vi "Send SetSlitwidth.vi"(7 "Message Priority (Normal)":T2=enum."Normal", 8 "error in (no error)":errorcluster, 9 "Slitwidth":u16, 10 "Slit":T1(ring), 11 "Message Enqueuer":refnum<class "Message Enqueuer.lvclass">) -> (0 "error out":errorcluster, 3 "Message Enqueuer out":refnum<class "Message Enqueuer.lvclass">)   [LabVIEW 2023, in "Spectrometer Library.lvlib" / "SpectrometerInterface.lvlib" / "SetSlitwidth Msg.lvclass"]
doc: "This VI sends the message to an actor."
uses:
  SetSlitwidth Msg.lvclass
  <vilib>/ActorFramework/Message Enqueuer/Message Enqueuer.lvclass
  <vilib>/ActorFramework/Message Enqueuer/Message Priority.ctl
  C:/Program Files/National Instruments/LabVIEW 2023/vi.lib/ActorFramework/Message/Message.lvclass
  SetSlitwidth Msg.lvclass/SetSlitwidth Msg.ctl
  <vilib>/ActorFramework/Message Enqueuer/Message Enqueuer.lvclass/Message Enqueuer.ctl
  <vilib>/ActorFramework/Message Priority Queue/Priority Enqueue.vi
  C:/Users/quantum/Documents/LVDAQ/Interfaces/AbstractInstrumentClasses/Spectrometers_LV/Spectrometer Messages/SetSlitwidth Msg/SetSlitwidth Msg.lvclass
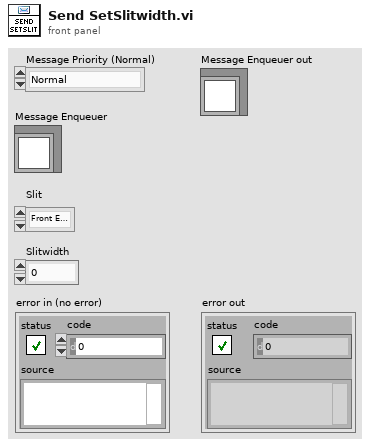
[diagram p1: front panel]
types:
  T1 = enum16{"Front Entrance", "Side Entrance", "Front Exit", "Side Exit"}
  T2 = typedef "Actor Framework.lvlib/Message Enqueuer.lvclass/Message Priority.ctl" = enum16{"Low", "Normal", "High"}
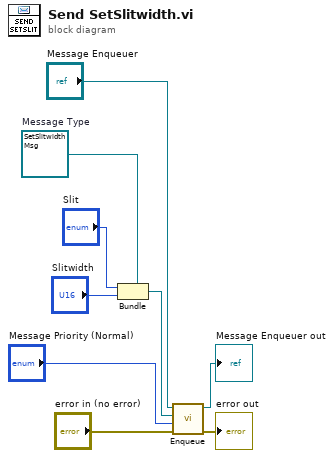
[diagram p0: block diagram]
diagram:
  w6 = refnum<class "SetSlitwidth Msg.lvclass"> refnum  # Message Type
  n1 = Bundle(cluster=w6, "Slit", "Slitwidth") -> (w5:refnum<class "SetSlitwidth Msg.lvclass">)
  n2 = call <vilib>:"Enqueue.vi"("error in (no error)"="error in (no error)", "Message Priority (Normal)"="Message Priority (Normal)", "Message"=w5, "Message Enqueuer in"="Message Enqueuer") -> ("error out"=→"error out":errorcluster, "Message Enqueuer in"=→"Message Enqueuer out":refnum<class "Message Enqueuer.lvclass">)  [unwired: 6 in]
